vi "Close Diagnostics File.vi"(8 "error in":errorcluster, 11 "diagnostics file":refnum<file>) -> (0 "error out":errorcluster, 3 "not a file refnum":refnum<file>)   [LabVIEW 2021, in "Diagnostics.lvlib"]
uses:
  Diagnostics.lvlib
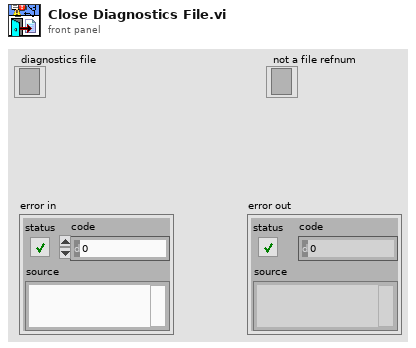
[diagram p1: front panel]
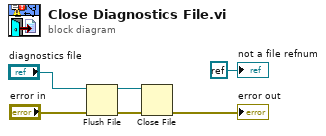
[diagram p0: block diagram]
diagram:
  n1 = Flush File(refnum="diagnostics file", error in="error in") -> (refnum out=w3:refnum<file>, error out=w1:errorcluster)
  n2 = Close File(refnum=w3, error in=w1) -> (error out=→"error out":errorcluster)  [unwired: 1 out]
  "not a file refnum" <- refnum<k0> refnum
